vi "Write Roles.vi"(8 "error in (no error)":errorcluster, 10 "Roles":T1, 11 "NormalDefensiveWithDuelistPlay in":refnum<class "NormalDefensiveWithDuelistPlay.lvclass">) -> (0 "error out":errorcluster, 3 "NormalDefensiveWithDuelistPlay out":refnum<class "NormalDefensiveWithDuelistPlay.lvclass">)   [LabVIEW 2023, in "NormalDefensiveWithDuelistPlay.lvclass"]
uses:
  NormalDefensiveWithDuelistPlay.lvclass
  DefenderAreaRole_class/DefenderAreaRole.lvclass
  DuelistRole_class/DuelistRole.lvclass
  NormalDefensiveWithDuelistPlay.lvclass/NormalDefensiveWithDuelistPlay.ctl
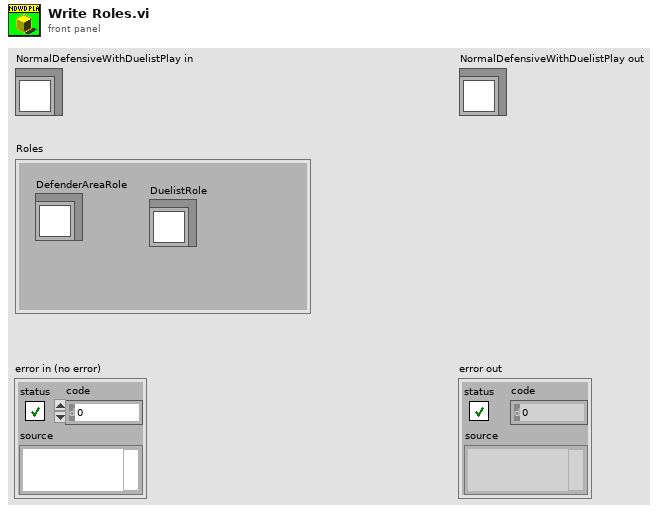
[diagram p1: front panel]
types:
  T1 = cluster{"DefenderAreaRole":refnum<class "DefenderAreaRole.lvclass">, "DuelistRole":refnum<class "DuelistRole.lvclass">}
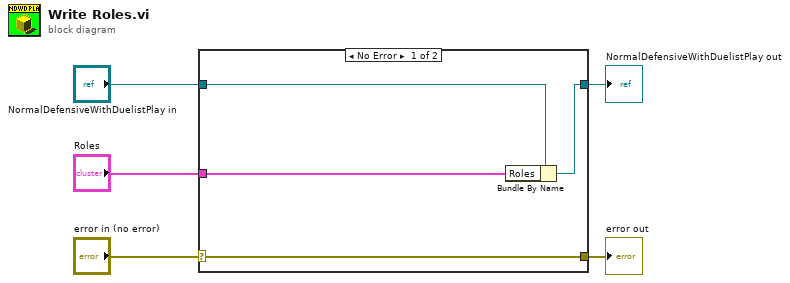
[diagram p0: block diagram]
diagram:
  n1 = case shown="No Error" "error in (no error)" {
    selector: "error in (no error)" -> [w9 w10]
    tunnel: [w9 w10] -> w4
    tunnel: [w7 w11] -> w2
    tunnel: "NormalDefensiveWithDuelistPlay in" -> [w8 w11]
    tunnel: "Roles" -> [w6 _]
    frame No Error {
      n2 = Bundle By Name(cluster=w8, "Roles"=w6) -> (w7:refnum<class "NormalDefensiveWithDuelistPlay.lvclass">)
    }
    frame Error {
    }
  }
  "error out" <- w4
  "NormalDefensiveWithDuelistPlay out" <- w2
